vi "Version 1_Write PID Settings.vi"(7 "Address (A)":string="A", 8 "error in":errorcluster, 9 "PID Loop Settings (\"Valve Amount\" no longer\nselectable, since it should not be altered)":T1={"P Gain"=0, "PID Type"=enum."PDF", "D Gain"=0, "I Gain"=0, "Valve Amount"=enum."Dual Valve"}, 11 "VISA Session In":refnum<visa-resource-name>="Alicat") -> (0 "error out":errorcluster, 3 "VISA Session Out":refnum<visa-resource-name>)   [LabVIEW 2016]
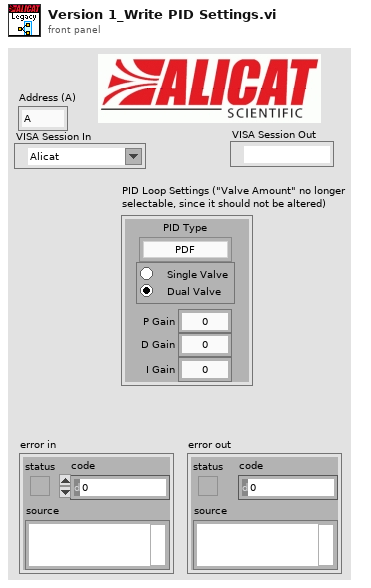
[diagram p1: front panel]
types:
  T1 = cluster{"P Gain":u16, "PID Type":enum8{"PDF", "PD2I"}, "D Gain":u16, "I Gain":u16, "Valve Amount":enum32{"Single Valve", "Dual Valve"}}
  T2 = cluster{"PID Type":enum8{"PDF", "PD2I"}, "Valve Offset":i32}
  T3 = cluster{"P Gain":i32, "D Gain":i32, "I Gain":i32}
  T4 = cluster{"Valve Amount":enum8{"Single Valve", "Dual Valve"}, "PID Type":enum8{"PDF", "PD2I"}, "Valve Offset":i32, "P Gain":i32, "D Gain":i32, "I Gain":i32}
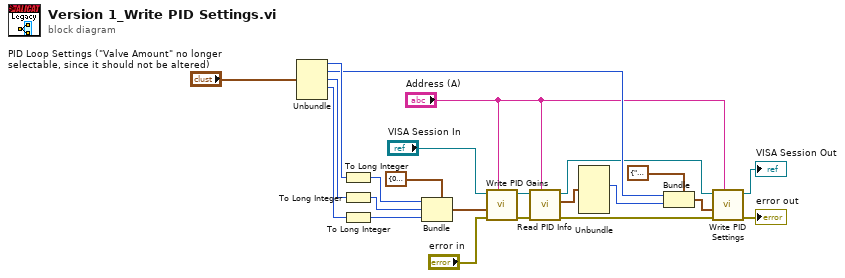
[diagram p0: block diagram]
diagram:
  n1 = Unbundle("PID Loop Settings (\"Valve Amount\" no longer\nselectable, since it should not be altered)") -> ("P Gain"=w14:u16, "PID Type"=w9:enum8{"PDF", "PD2I"}, "D Gain"=w13:u16, "I Gain"=w12:u16)  [unwired: 1 out]
  n2 = To Long Integer(number=w14) -> (32bit integer=w17:i32)
  n3 = To Long Integer(number=w13) -> (32bit integer=w15:i32)
  n4 = To Long Integer(number=w12) -> (32bit integer=w16:i32)
  n5 = Bundle(cluster=T3 {"P Gain"=0, "D Gain"=0, "I Gain"=0} ("PID Gain Settings"), "P Gain"=w17, "D Gain"=w15, "I Gain"=w16) -> (w1:T3)
  n6 = call "Write PID Gains.vi"("VISA Session In"="VISA Session In", "PID Gain Settings"=w1, "error in"="error in", "Unit ID (A)"="Address (A)") -> ("VISA Session Out"=w7:refnum<visa-resource-name>, "error out"=w8:errorcluster)  [unwired: 5 in]
  n7 = call "Read PID Info.vi"("VISA Session In"=w7, "error in"=w8, "Unit ID (A)"="Address (A)") -> ("VISA Session Out"=w2:refnum<visa-resource-name>, "PID Settings"=w5:T4, "error out"=w3:errorcluster)  [unwired: 5 in]
  n8 = Unbundle(w5) -> ("Valve Offset"=w4:i32)  [unwired: 5 out]
  n9 = Bundle(cluster=T2 {"PID Type"=enum."PDF", "Valve Offset"=18000} ("PID Loop Settings"), "PID Type"=w9, "Valve Offset"=w4) -> (w10:T2)
  n10 = call "Write PID Settings.vi"("VISA Session In"=w2, "PID Loop Settings"=w10, "error in"=w3, "Unit ID (A)"="Address (A)") -> ("VISA Session Out"=→"VISA Session Out":refnum<visa-resource-name>, "error out"=→"error out":errorcluster)  [unwired: 5 in]
